vi "Lab Panel V6.00.vi"() -> ()   [LabVIEW 2017] (continued)
                          tunnel: w826 -> [_ w839]
                          tunnel: w824 -> [_ w838]
                          frame False {
                            w836 = FALSE
                            n593 = local write "RUN LAB01-1"(w836) -> ()
                            n594 = local write "run lab01-1"(w836) -> ()
                          }
                          frame True {
                            n595 = stacked-sequence {
                              seq-local: [w849 _ _ _ _] -> [_ w870 _ _ _]
                              tunnel: w848 -> [w854 _ _ _ _]
                              tunnel: w847 -> [w850 _ _ _ _]
                              tunnel: w846 -> [w864 _ _ _ _]
                              tunnel: w845 -> [w857 _ _ _ _]
                              tunnel: w844 -> [w852 _ _ _ _]
                              tunnel: [_ w871 _ _ _] -> w843
                              tunnel: w842 -> [_ _ _ w892 _]
                              tunnel: w841 -> [_ _ _ w902 _]
                              tunnel: w840 -> [_ _ _ w901 _]
                              tunnel: w839 -> [_ _ _ _ _]
                              tunnel: w838 -> [_ _ _ _ w908]
                              frame #0 {
                                w851 = "\\"
                                n596 = case shown="\"CHART TEST\", Default" w864 {
                                tunnel: ["L01-1-CHART TEST-" "L01-1-CYCLE TEST-" "L01-1-T-RISE TEST-"] -> w860
                                frame "CHART TEST", Default {
                                }
                                frame "CYCLE TEST" {
                                }
                                frame "T-RISE TEST" {
                                }
                                }
                                n597 = local read "SET LAB01-1"() -> (w859:T6)
                                n598 = Unbundle By Name(w859) -> ("DESCRIPTION"=w858:string)
                                n599 = Concatenate Strings(w854, "\\", w852, w851, w850, w851) -> (w861:string)
                                n600 = String To Path(string=w861) -> (path=w863:path)
                                n601 = Concatenate Strings(w861, w860, w858, "-", w857, ".tdms") -> (w849:string)
                                n602 = Create Folder(path (use dialog)=w863) -> (error out=w862:errorcluster)  [unwired: 2 in, 2 out]
                                n603 = call <vilib>:"Clear Errors.vi"("error in (no error)"=w862) -> ()  [unwired: 5 in, 2 out]
                                n604 = global write "Global 1.vi" "LAB01-1 FILE"(w849) -> ()
                              }
                              frame #1 {
                                (unwired) FALSE
                                n605 = String To Path(string=w870) -> (path=w868:path)
                                n606 = TDMS Open(6:FALSE, 10:T22."create or replace" ("operation (0:open)"), 11:w868) -> (0:w871:errorcluster, 3:→"TDMS LAB01-1":refnum<k34>)  [unwired: 4 in]
                              }
                              frame #2 {
                                n607 = local read "TDMS LAB01-1"() -> (w890:refnum<k34>)
                                n608 = local read "SET LAB01-1"() -> (w879:T6)
                                n609 = Build Array("Testers Name", "Description", "Set Test Cycles", "T-Rise minutes", "T-Rise Deg C") -> (w880:string[])
                                n610 = Unbundle(w879) -> ("NAME"=w878:string, "DESCRIPTION"=w877:string, "CYCLES"=w876:dbl, "T-RISE mins"=w875:dbl, "T-RISE deg C"=w874:dbl)
                                n611 = Number To Decimal String(number=w876) -> (decimal integer string=w889:string)  [unwired: 1 in]
                                n612 = Number To Decimal String(number=w875) -> (decimal integer string=w888:string)  [unwired: 1 in]
                                n613 = Number To Decimal String(number=w874) -> (decimal integer string=w887:string)  [unwired: 1 in]
                                n614 = Build Array(w878, w877, w889, w888, w887) -> (w886:string[])
                                n615 = TDMS Set Properties(5:w886, 7:w880, 11:w890) -> ()  [unwired: 3 in, 4 out]
                              }
                              frame #3 {
                                n616 = local read "DISP LAB01-1"() -> (w900:T4)
                                n617 = Concatenate Strings("LAB01-1  ", w892) -> (w891:string)
                                n618 = Two Button Dialog(message=w891, 1:w901, 2:w902) -> (T button?=w894:bool)
                                n619 = case shown="True" w894 {
                                tunnel: w900 -> [w905 w906]
                                tunnel: [w905 w906] -> w899
                                tunnel: [w904 w907] -> w898
                                tunnel: [w903 w907] -> w897
                                frame False {
                                n620 = Unbundle(w905) -> ("CYCLE"=w904:dbl, "MINS"=w903:dbl)  [unwired: 1 out]
                                }
                                frame True {
                                w907 = 0.0
                                }
                                }
                                n621 = Bundle(cluster=w899, "CYCLE"=w898, "MINS"=w897, "STATUS"="RUN") -> (w896:T4)
                                n622 = local write "DISP LAB01-1"(w896) -> ()
                              }
                              frame #4 {
                                n623 = local read "TEMP START LAB01-1"() -> (w910:cluster{"TL":dbl, "TN":dbl})
                                n624 = Bundle(cluster=w910, "TL"=w908, "TN"=w908) -> (w909:cluster{"TL":dbl, "TN":dbl})
                                n625 = local write "TEMP START LAB01-1"(w909) -> ()
                              }
                            }
                          }
                        }
                      }
                    }
                  }
                }
              }
              event "RUN LAB01-2": Value Change {
                n626 = event-data() -> ("NewVal"=w915:bool)  [unwired: 1 in, 5 out]
                n627 = local write "run lab01-2"(w915) -> ()
                n628 = case shown="True" w915 {
                  tunnel: w921 -> [_ w959]
                  tunnel: w920 -> [_ w958]
                  tunnel: w918 -> [w923 w957]
                  tunnel: w919 -> [_ w956]
                  tunnel: w917 -> [_ w955]
                  tunnel: [w922 w954] -> w916
                  tunnel: w914 -> [_ w953]
                  tunnel: w913 -> [_ w952]
                  tunnel: w912 -> [_ w951]
                  tunnel: w911 -> [_ w949]
                  frame False {
                    # "stop test"
                    n629 = stacked-sequence {
                      tunnel: w923 -> [w932 _]
                      tunnel: [w924 _] -> w922
                      frame #0 {
                        n630 = local read "DISP LAB01-2"() -> (w931:T4)
                        n631 = Unbundle(w931) -> ("CYCLE"=w929:dbl, "MINS"=w930:dbl)  [unwired: 1 out]
                        n632 = case shown="\"CHART TEST\", Default" w932 {
                          tunnel: w930 -> [_ _ w939]
                          tunnel: w929 -> [w937 w938 _]
                          tunnel: [w937 w938 w939] -> w928
                          frame "CHART TEST", Default {
                          }
                          frame "CYCLE TEST" {
                          }
                          frame "T-RISE TEST" {
                          }
                        }
                        n633 = local read "TDMS LAB01-2"() -> (w936:refnum<k34>)
                        n634 = Build Array("STOPPED") -> (w933:string[])
                        n635 = Build Array(w928) -> (w927:dbl[])
                        n636 = TDMS Write(0:w936, 5:"TEST RESULT", 7:w933, 9:w927) -> (4:w925:refnum<k34>, 15:w926:errorcluster)  [unwired: 2 in, 2 out]
                        n637 = TDMS Close(8:w926, 11:w925) -> (0:w924:errorcluster)  [unwired: 1 out]
                      }
                      frame #1 {
                        n638 = local read "DISP LAB01-2"() -> (w943:T4)
                        n639 = stacked-sequence {
                          tunnel: "LAB01-2" -> [w945 w947]
                          frame #0 {
                            n640 = call "sub vi - defrag tdms v1.vi"("panel id"=w945) -> ("error out"=w944:errorcluster)  [unwired: 10 in]
                            n641 = local write "data file error"(w944) -> ()
                          }
                          frame #1 {
                            n642 = call "Save data file (stop) v3.vi"("panel id"=w947) -> ("network file save error"=w946:errorcluster)  [unwired: 9 in, 1 out]
                            n643 = local write "RESULT LAB01-2"(FALSE) -> ()
                            n644 = local write "data file error"(w946) -> ()
                          }
                        }
                        n645 = Bundle(cluster=w943, "STATUS"="STOP") -> (w941:T4)  [unwired: 2 in]
                        n646 = local write "DISP LAB01-2"(w941) -> ()
                      }
                    }
                  }
                  frame True {
                    n647 = local read "SIG LAB01-2"() -> (w950:T2)
                    n648 = stacked-sequence {
                      seq-local: [w961 _] -> [_ w965]
                      tunnel: w959 -> [_ w975]
                      tunnel: w958 -> [_ w974]
                      tunnel: w957 -> [_ w973]
                      tunnel: w956 -> [_ w972]
                      tunnel: w955 -> [_ w971]
                      tunnel: [_ w970] -> w954
                      tunnel: w953 -> [_ w969]
                      tunnel: w952 -> [_ w968]
                      tunnel: w951 -> [_ w967]
                      tunnel: w950 -> [w960 w966]
                      tunnel: w949 -> [_ w964]
                      frame #0 {
                        n649 = Unbundle(w960) -> ("AMPS"=w963:dbl)  [unwired: 4 out]
                        n650 = call "Check For Amps on v1.vi"("ID"="LAB01-2", "amps"=w963) -> ("amps"=w961:bool)  [unwired: 9 in]
                      }
                      frame #1 {
                        n651 = case shown="True" w965 {
                          tunnel: w975 -> [_ w988]
                          tunnel: w974 -> [_ w987]
                          tunnel: w973 -> [_ w986]
                          tunnel: w972 -> [_ w985]
                          tunnel: w971 -> [_ w984]
                          tunnel: [errorcluster {"status"=FALSE, "code"=0, "source"=""} ("error out") w983] -> w970
                          tunnel: w969 -> [_ w982]
                          tunnel: w968 -> [_ w981]
                          tunnel: w967 -> [_ w980]
                          tunnel: w966 -> [_ w979]
                          tunnel: w964 -> [_ w978]
                          frame False {
                            w976 = FALSE
                            n652 = local write "RUN LAB01-2"(w976) -> ()
                            n653 = local write "run lab01-2"(w976) -> ()
                          }
                          frame True {
                            n654 = stacked-sequence {
                              seq-local: [w989 _ _ _ _] -> [_ w1013 _ _ _]
                              tunnel: w988 -> [w994 _ _ _ _]
                              tunnel: w987 -> [w991 _ _ _ _]
                              tunnel: w986 -> [w1004 _ _ _ _]
                              tunnel: w985 -> [w997 _ _ _ _]
                              tunnel: w984 -> [w992 _ _ _ _]
                              tunnel: [_ w1008 _ _ _] -> w983
                              tunnel: w982 -> [_ _ _ w1035 _]
                              tunnel: w981 -> [_ _ _ w1034 _]
                              tunnel: w980 -> [_ _ _ w1033 _]
                              tunnel: w979 -> [_ _ _ _ _]
                              tunnel: w978 -> [_ _ _ _ w1048]
                              frame #0 {
                                w990 = "\\"
                                n655 = local read "SET LAB01-2"() -> (w999:T5)
                                n656 = case shown="\"CYCLE TEST\"" w1004 {
                                tunnel: ["L01-2-CHART TEST-" "L01-2-CYCLE TEST-" "L01-2-T-RISE TEST-"] -> w1000
                                frame "CHART TEST", Default {
                                }
                                frame "CYCLE TEST" {
                                }
                                frame "T-RISE TEST" {
                                }
                                }
                                n657 = Unbundle(w999) -> ("DESCRIPTION"=w998:string)  [unwired: 4 out]
                                n658 = Concatenate Strings(w994, "\\", w992, w990, w991, w990) -> (w1001:string)
                                n659 = String To Path(string=w1001) -> (path=w1003:path)
                                n660 = Concatenate Strings(w1001, w1000, w998, "-", w997, ".tdms") -> (w989:string)
                                n661 = Create Folder(path (use dialog)=w1003) -> (error out=w1002:errorcluster)  [unwired: 2 in, 2 out]
                                n662 = call <vilib>:"Clear Errors.vi"("error in (no error)"=w1002) -> ()  [unwired: 5 in, 2 out]
                                n663 = global write "Global 1.vi" "LAB01-2 FILE"(w989) -> ()
                              }
                              frame #1 {
                                (unwired) FALSE
                                n664 = String To Path(string=w1013) -> (path=w1009:path)
                                n665 = TDMS Open(6:FALSE, 10:T22."create or replace" ("operation (0:open)"), 11:w1009) -> (0:w1008:errorcluster, 3:→"TDMS LAB01-2":refnum<k34>)  [unwired: 4 in]
                              }
                              frame #2 {
                                n666 = local read "SET LAB01-2"() -> (w1019:T5)
                                n667 = local read "TDMS LAB01-2"() -> (w1030:refnum<k34>)
                                n668 = Build Array("Testers Name", "Description", "Set Test Cycles", "T-Rise minutes", "T-Rise Deg C") -> (w1020:string[])
                                n669 = Unbundle(w1019) -> ("NAME"=w1018:string, "DESCRIPTION"=w1017:string, "CYCLES"=w1016:dbl, "T-RISE mins"=w1015:dbl, "T-RISE deg C"=w1014:dbl)
                                n670 = Number To Decimal String(number=w1016) -> (decimal integer string=w1029:string)  [unwired: 1 in]
                                n671 = Number To Decimal String(number=w1015) -> (decimal integer string=w1028:string)  [unwired: 1 in]
                                n672 = Number To Decimal String(number=w1014) -> (decimal integer string=w1027:string)  [unwired: 1 in]
                                n673 = Build Array(w1018, w1017, w1029, w1028, w1027) -> (w1026:string[])
                                n674 = TDMS Set Properties(5:w1026, 7:w1020, 11:w1030) -> ()  [unwired: 3 in, 4 out]
                              }
                              frame #3 {
                                n675 = local read "DISP LAB01-2"() -> (w1032:T4)
                                n676 = Concatenate Strings("LAB01-2  ", w1035) -> (w1036:string)
                                n677 = Two Button Dialog(message=w1036, 1:w1033, 2:w1034) -> (T button?=w1038:bool)
                                n678 = case shown="True" w1038 {
                                tunnel: w1032 -> [w1045 w1046]
                                tunnel: [w1045 w1046] -> w1042
                                tunnel: [w1044 w1047] -> w1041
                                tunnel: [w1043 w1047] -> w1040
                                frame False {
                                n679 = Unbundle(w1045) -> ("CYCLE"=w1044:dbl, "MINS"=w1043:dbl)  [unwired: 1 out]
                                }
                                frame True {
                                w1047 = 0.0
                                }
                                }
                                n680 = Bundle(cluster=w1042, "CYCLE"=w1041, "MINS"=w1040, "STATUS"="RUN") -> (w1031:T4)
                                n681 = local write "DISP LAB01-2"(w1031) -> ()
                              }
                              frame #4 {
                                n682 = local read "TEMP START LAB01-2"() -> (w1050:cluster{"TL":dbl, "TN":dbl})
                                n683 = Bundle(cluster=w1050, "TL"=w1048, "TN"=w1048) -> (w1049:cluster{"TL":dbl, "TN":dbl})
                                n684 = local write "TEMP START LAB01-2"(w1049) -> ()
                              }
                            }
                          }
                        }
                      }
                    }
                  }
                }
              }
              event "RUN LAB02-1": Value Change {
                n685 = event-data() -> ("NewVal"=w1056:bool)  [unwired: 1 in, 5 out]
                n686 = local read "SIG LAB02-1"() -> (w1052:T2)
                n687 = case shown="True" w1056 {
                  tunnel: w1062 -> [_ w1100]
                  tunnel: w1061 -> [_ w1099]
                  tunnel: w1059 -> [w1064 w1098]
                  tunnel: w1060 -> [_ w1097]
                  tunnel: w1058 -> [_ w1096]
                  tunnel: [w1063 w1095] -> w1057
                  tunnel: w1055 -> [_ w1094]
                  tunnel: w1054 -> [_ w1093]
                  tunnel: w1053 -> [_ w1092]
                  tunnel: w1052 -> [_ w1091]
                  tunnel: w1051 -> [_ w1090]
                  frame False {
                    # "stop test"
                    n688 = stacked-sequence {
                      tunnel: w1064 -> [w1073 _]
                      tunnel: [w1065 _] -> w1063
                      frame #0 {
                        n689 = local read "DISP LAB02-1"() -> (w1072:T4)
                        n690 = Unbundle(w1072) -> ("CYCLE"=w1070:dbl, "MINS"=w1071:dbl)  [unwired: 1 out]
                        n691 = case shown="\"CYCLE TEST\"" w1073 {
                          tunnel: w1071 -> [_ _ w1080]
                          tunnel: w1070 -> [w1078 w1079 _]
                          tunnel: [w1078 w1079 w1080] -> w1069
                          frame "CHART TEST", Default {
                          }
                          frame "CYCLE TEST" {
                          }
                          frame "T-RISE TEST" {
                          }
                        }
                        n692 = local read "TDMS LAB02-1"() -> (w1077:refnum<k34>)
                        n693 = Build Array("STOPPED") -> (w1074:string[])
                        n694 = Build Array(w1069) -> (w1068:dbl[])
                        n695 = TDMS Write(0:w1077, 5:"TEST RESULT", 7:w1074, 9:w1068) -> (4:w1066:refnum<k34>, 15:w1067:errorcluster)  [unwired: 2 in, 2 out]
                        n696 = TDMS Close(8:w1067, 11:w1066) -> (0:w1065:errorcluster)  [unwired: 1 out]
                      }
                      frame #1 {
                        n697 = local read "DISP LAB02-1"() -> (w1084:T4)
                        n698 = stacked-sequence {
                          tunnel: "LAB02-1" -> [w1086 w1088]
                          frame #0 {
                            n699 = call "sub vi - defrag tdms v1.vi"("panel id"=w1086) -> ("error out"=w1085:errorcluster)  [unwired: 10 in]
                            n700 = local write "data file error"(w1085) -> ()
                          }
                          frame #1 {
                            n701 = local write "RESULT LAB02-1"(FALSE) -> ()
                            n702 = call "Save data file (stop) v3.vi"("panel id"=w1088) -> ("network file save error"=w1087:errorcluster)  [unwired: 9 in, 1 out]
                            n703 = local write "data file error"(w1087) -> ()
                          }
                        }
                        n704 = Bundle(cluster=w1084, "STATUS"="STOP") -> (w1082:T4)  [unwired: 2 in]
                        n705 = local write "DISP LAB02-1"(w1082) -> ()
                      }
                    }
                  }
                  frame True {
                    n706 = stacked-sequence {
                      seq-local: [w1102 _] -> [_ w1106]
                      tunnel: w1100 -> [_ w1116]
                      tunnel: w1099 -> [_ w1115]
                      tunnel: w1098 -> [_ w1114]
                      tunnel: w1097 -> [_ w1113]
                      tunnel: w1096 -> [_ w1112]
                      tunnel: [_ w1111] -> w1095
                      tunnel: w1094 -> [_ w1110]
                      tunnel: w1093 -> [_ w1109]
                      tunnel: w1092 -> [_ w1108]
                      tunnel: w1091 -> [w1101 w1107]
                      tunnel: w1090 -> [_ w1105]
                      frame #0 {
                        n707 = Unbundle(w1101) -> ("AMPS"=w1104:dbl)  [unwired: 4 out]
                        n708 = call "Check For Amps on v1.vi"("ID"="LAB02-1", "amps"=w1104) -> ("amps"=w1102:bool)  [unwired: 9 in]
                      }
                      frame #1 {
                        n709 = case shown="True" w1106 {
                          tunnel: w1116 -> [_ w1129]
                          tunnel: w1115 -> [_ w1128]
                          tunnel: w1114 -> [_ w1127]
                          tunnel: w1113 -> [_ w1126]
                          tunnel: w1112 -> [_ w1125]
                          tunnel: [errorcluster {"status"=FALSE, "code"=0, "source"=""} ("error out") w1124] -> w1111
                          tunnel: w1110 -> [_ w1123]
                          tunnel: w1109 -> [_ w1122]
                          tunnel: w1108 -> [_ w1121]
                          tunnel: w1107 -> [_ w1120]
                          tunnel: w1105 -> [_ w1119]
                          frame False {
                            w1118 = FALSE
                            n710 = local write "RUN LAB02-1"(w1118) -> ()
                            n711 = local write "run lab02-1"(w1118) -> ()
                          }
                          frame True {
                            n712 = stacked-sequence {
                              seq-local: [w1130 _ _ _ _] -> [_ w1154 _ _ _]
                              tunnel: w1129 -> [w1135 _ _ _ _]
                              tunnel: w1128 -> [w1132 _ _ _ _]
                              tunnel: w1127 -> [w1145 _ _ _ _]
                              tunnel: w1126 -> [w1138 _ _ _ _]
                              tunnel: w1125 -> [w1133 _ _ _ _]
                              tunnel: [_ w1149 _ _ _] -> w1124
                              tunnel: w1123 -> [_ _ _ w1175 _]
                              tunnel: w1122 -> [_ _ _ w1174 _]
                              tunnel: w1121 -> [_ _ _ w1173 _]
                              tunnel: w1120 -> [_ _ _ _ _]
                              tunnel: w1119 -> [_ _ _ _ w1189]
                              frame #0 {
                                w1131 = "\\"
                                n713 = local read "SET LAB02-1"() -> (w1140:T5)
                                n714 = case shown="\"CYCLE TEST\"" w1145 {
                                tunnel: ["L02-1-CHART TEST-" "L02-1-CYCLE TEST-" "L02-1-T-RISE TEST-"] -> w1141
                                frame "CHART TEST", Default {
                                }
                                frame "CYCLE TEST" {
                                }
                                frame "T-RISE TEST" {
                                }
                                }
                                n715 = Unbundle(w1140) -> ("DESCRIPTION"=w1139:string)  [unwired: 4 out]
                                n716 = Concatenate Strings(w1135, "\\", w1133, w1131, w1132, w1131) -> (w1142:string)
                                n717 = String To Path(string=w1142) -> (path=w1144:path)
                                n718 = Concatenate Strings(w1142, w1141, w1139, "-", w1138, ".tdms") -> (w1130:string)
                                n719 = Create Folder(path (use dialog)=w1144) -> (error out=w1143:errorcluster)  [unwired: 2 in, 2 out]
                                n720 = global write "Global 1.vi" "LAB02-1 FILE"(w1130) -> ()
                                n721 = call <vilib>:"Clear Errors.vi"("error in (no error)"=w1143) -> ()  [unwired: 5 in, 2 out]
                              }
                              frame #1 {
                                (unwired) FALSE
                                n722 = String To Path(string=w1154) -> (path=w1150:path)
                                n723 = TDMS Open(6:FALSE, 10:T22."create or replace" ("operation (0:open)"), 11:w1150) -> (0:w1149:errorcluster, 3:→"TDMS LAB02-1":refnum<k34>)  [unwired: 4 in]
                              }
                              frame #2 {
                                n724 = local read "SET LAB02-1"() -> (w1160:T5)
                                n725 = local read "TDMS LAB02-1"() -> (w1171:refnum<k34>)
                                n726 = Build Array("Testers Name", "Description", "Set Test Cycles", "T-Rise minutes", "T-Rise Deg C") -> (w1161:string[])
                                n727 = Unbundle(w1160) -> ("NAME"=w1159:string, "DESCRIPTION"=w1158:string, "CYCLES"=w1157:dbl, "T-RISE mins"=w1156:dbl, "T-RISE deg C"=w1155:dbl)
                                n728 = Number To Decimal String(number=w1157) -> (decimal integer string=w1170:string)  [unwired: 1 in]
                                n729 = Number To Decimal String(number=w1156) -> (decimal integer string=w1169:string)  [unwired: 1 in]
                                n730 = Number To Decimal String(number=w1155) -> (decimal integer string=w1168:string)  [unwired: 1 in]
                                n731 = Build Array(w1159, w1158, w1170, w1169, w1168) -> (w1167:string[])
                                n732 = TDMS Set Properties(5:w1167, 7:w1161, 11:w1171) -> ()  [unwired: 3 in, 4 out]
                              }
                              frame #3 {
                                n733 = local read "DISP LAB02-1"() -> (w1176:T4)
                                n734 = Concatenate Strings("LAB02-1  ", w1175) -> (w1177:string)
                                n735 = Two Button Dialog(message=w1177, 1:w1173, 2:w1174) -> (T button?=w1179:bool)
                                n736 = case shown="True" w1179 {
                                tunnel: w1176 -> [w1186 w1187]
                                tunnel: [w1186 w1187] -> w1183
                                tunnel: [w1185 w1188] -> w1182
                                tunnel: [w1184 w1188] -> w1181
                                frame False {
                                n737 = Unbundle(w1186) -> ("CYCLE"=w1185:dbl, "MINS"=w1184:dbl)  [unwired: 1 out]
                                }
                                frame True {
                                w1188 = 0.0
                                }
                                }
                                n738 = Bundle(cluster=w1183, "CYCLE"=w1182, "MINS"=w1181, "STATUS"="RUN") -> (w1172:T4)
                                n739 = local write "DISP LAB02-1"(w1172) -> ()
                              }
                              frame #4 {
                                n740 = local read "TEMP START LAB02-1"() -> (w1191:cluster{"TL":dbl, "TN":dbl})
                                n741 = Bundle(cluster=w1191, "TL"=w1189, "TN"=w1189) -> (w1190:cluster{"TL":dbl, "TN":dbl})
                                n742 = local write "TEMP START LAB02-1"(w1190) -> ()
                              }
                            }
                          }
                        }
                      }
                    }
                  }
                }
                n743 = local write "run lab02-1"(w1056) -> ()
              }
              event "RUN LAB02-2": Value Change {
                n744 = event-data() -> ("NewVal"=w1196:bool)  [unwired: 1 in, 5 out]
                n745 = local write "run lab02-2"(w1196) -> ()
                n746 = case shown="True" w1196 {
                  tunnel: w1202 -> [_ w1240]
                  tunnel: w1201 -> [_ w1239]
                  tunnel: w1199 -> [w1204 w1238]
                  tunnel: w1200 -> [_ w1237]
                  tunnel: w1198 -> [_ w1236]
                  tunnel: [w1203 w1235] -> w1197
                  tunnel: w1195 -> [_ w1234]
                  tunnel: w1194 -> [_ w1233]
                  tunnel: w1193 -> [_ w1232]
                  tunnel: w1192 -> [_ w1230]
                  frame False {
                    # "stop test"
                    n747 = stacked-sequence {
                      tunnel: w1204 -> [w1213 _]
                      tunnel: [w1205 _] -> w1203
                      frame #0 {
                        n748 = local read "DISP LAB02-2"() -> (w1212:T4)
                        n749 = Unbundle(w1212) -> ("CYCLE"=w1210:dbl, "MINS"=w1211:dbl)  [unwired: 1 out]
                        n750 = case shown="\"CYCLE TEST\"" w1213 {
                          tunnel: w1211 -> [_ _ w1220]
                          tunnel: w1210 -> [w1218 w1219 _]
                          tunnel: [w1218 w1219 w1220] -> w1209
                          frame "CHART TEST", Default {
                          }
                          frame "CYCLE TEST" {
                          }
                          frame "T-RISE TEST" {
                          }
                        }
                        n751 = local read "TDMS LAB02-2"() -> (w1217:refnum<k34>)
                        n752 = Build Array("STOPPED") -> (w1214:string[])
                        n753 = Build Array(w1209) -> (w1208:dbl[])
                        n754 = TDMS Write(0:w1217, 5:"TEST RESULT", 7:w1214, 9:w1208) -> (4:w1206:refnum<k34>, 15:w1207:errorcluster)  [unwired: 2 in, 2 out]
                        n755 = TDMS Close(8:w1207, 11:w1206) -> (0:w1205:errorcluster)  [unwired: 1 out]
                      }
                      frame #1 {
                        n756 = local read "DISP LAB02-2"() -> (w1224:T4)
                        n757 = stacked-sequence {
                          tunnel: "LAB02-2" -> [w1226 w1228]
                          frame #0 {
                            n758 = call "sub vi - defrag tdms v1.vi"("panel id"=w1226) -> ("error out"=w1225:errorcluster)  [unwired: 10 in]
                            n759 = local write "data file error"(w1225) -> ()
                          }
                          frame #1 {
                            n760 = call "Save data file (stop) v3.vi"("panel id"=w1228) -> ("network file save error"=w1227:errorcluster)  [unwired: 9 in, 1 out]
                            n761 = local write "RESULT LAB02-2"(FALSE) -> ()
                            n762 = local write "data file error"(w1227) -> ()
                          }
                        }
                        n763 = Bundle(cluster=w1224, "STATUS"="STOP") -> (w1222:T4)  [unwired: 2 in]
                        n764 = local write "DISP LAB02-2"(w1222) -> ()
                      }
                    }
                  }
                  frame True {
                    n765 = local read "SIG LAB02-2"() -> (w1231:T2)
                    n766 = stacked-sequence {
                      seq-local: [w1242 _] -> [_ w1246]
                      tunnel: w1240 -> [_ w1256]
                      tunnel: w1239 -> [_ w1255]
                      tunnel: w1238 -> [_ w1254]
                      tunnel: w1237 -> [_ w1253]
                      tunnel: w1236 -> [_ w1252]
                      tunnel: [_ w1251] -> w1235
                      tunnel: w1234 -> [_ w1250]
                      tunnel: w1233 -> [_ w1249]
                      tunnel: w1232 -> [_ w1248]
                      tunnel: w1231 -> [w1241 w1247]
                      tunnel: w1230 -> [_ w1245]
                      frame #0 {
                        n767 = Unbundle(w1241) -> ("AMPS"=w1244:dbl)  [unwired: 4 out]
                        n768 = call "Check For Amps on v1.vi"("ID"="LAB02-2", "amps"=w1244) -> ("amps"=w1242:bool)  [unwired: 9 in]
                      }
                      frame #1 {
                        n769 = case shown="True" w1246 {
                          tunnel: w1256 -> [_ w1269]
                          tunnel: w1255 -> [_ w1268]
                          tunnel: w1254 -> [_ w1267]
                          tunnel: w1253 -> [_ w1266]
                          tunnel: w1252 -> [_ w1265]
                          tunnel: [errorcluster {"status"=FALSE, "code"=0, "source"=""} ("error out") w1264] -> w1251
                          tunnel: w1250 -> [_ w1263]
                          tunnel: w1249 -> [_ w1262]
                          tunnel: w1248 -> [_ w1261]
                          tunnel: w1247 -> [_ w1260]
                          tunnel: w1245 -> [_ w1259]
                          frame False {
                            w1257 = FALSE
                            n770 = local write "RUN LAB02-2"(w1257) -> ()
                            n771 = local write "run lab02-2"(w1257) -> ()
                          }
                          frame True {
                            n772 = stacked-sequence {
                              seq-local: [w1270 _ _ _ _] -> [_ w1294 _ _ _]
                              tunnel: w1269 -> [w1275 _ _ _ _]
                              tunnel: w1268 -> [w1272 _ _ _ _]
                              tunnel: w1267 -> [w1285 _ _ _ _]
                              tunnel: w1266 -> [w1278 _ _ _ _]
                              tunnel: w1265 -> [w1273 _ _ _ _]
                              tunnel: [_ w1289 _ _ _] -> w1264
                              tunnel: w1263 -> [_ _ _ w1315 _]
                              tunnel: w1262 -> [_ _ _ w1314 _]
                              tunnel: w1261 -> [_ _ _ w1313 _]
                              tunnel: w1260 -> [_ _ _ _ _]
                              tunnel: w1259 -> [_ _ _ _ w1329]
                              frame #0 {
                                w1271 = "\\"
                                n773 = local read "SET LAB02-2"() -> (w1280:T5)
                                n774 = case shown="\"CYCLE TEST\"" w1285 {
                                tunnel: ["L02-2-CHART TEST-" "L02-2-CYCLE TEST-" "L02-2-T-RISE TEST-"] -> w1281
                                frame "CHART TEST", Default {
                                }
                                frame "CYCLE TEST" {
                                }
                                frame "T-RISE TEST" {
                                }
                                }
                                n775 = Unbundle(w1280) -> ("DESCRIPTION"=w1279:string)  [unwired: 4 out]
                                n776 = Concatenate Strings(w1275, "\\", w1273, w1271, w1272, w1271) -> (w1282:string)
                                n777 = String To Path(string=w1282) -> (path=w1284:path)
                                n778 = Concatenate Strings(w1282, w1281, w1279, "-", w1278, ".tdms") -> (w1270:string)
                                n779 = Create Folder(path (use dialog)=w1284) -> (error out=w1283:errorcluster)  [unwired: 2 in, 2 out]
                                n780 = global write "Global 1.vi" "LAB02-2 FILE"(w1270) -> ()
                                n781 = call <vilib>:"Clear Errors.vi"("error in (no error)"=w1283) -> ()  [unwired: 5 in, 2 out]
                              }
                              frame #1 {
                                (unwired) FALSE
                                n782 = String To Path(string=w1294) -> (path=w1290:path)
                                n783 = TDMS Open(6:FALSE, 10:T22."create or replace" ("operation (0:open)"), 11:w1290) -> (0:w1289:errorcluster, 3:→"TDMS LAB02-2":refnum<k34>)  [unwired: 4 in]
                              }
                              frame #2 {
                                n784 = local read "SET LAB02-2"() -> (w1300:T5)
                                n785 = local read "TDMS LAB02-2"() -> (w1311:refnum<k34>)
                                n786 = Build Array("Testers Name", "Description", "Set Test Cycles", "T-Rise minutes", "T-Rise Deg C") -> (w1301:string[])
                                n787 = Unbundle(w1300) -> ("NAME"=w1299:string, "DESCRIPTION"=w1298:string, "CYCLES"=w1297:dbl, "T-RISE mins"=w1296:dbl, "T-RISE deg C"=w1295:dbl)
                                n788 = Number To Decimal String(number=w1297) -> (decimal integer string=w1310:string)  [unwired: 1 in]
                                n789 = Number To Decimal String(number=w1296) -> (decimal integer string=w1309:string)  [unwired: 1 in]
                                n790 = Number To Decimal String(number=w1295) -> (decimal integer string=w1308:string)  [unwired: 1 in]
                                n791 = Build Array(w1299, w1298, w1310, w1309, w1308) -> (w1307:string[])
                                n792 = TDMS Set Properties(5:w1307, 7:w1301, 11:w1311) -> ()  [unwired: 3 in, 4 out]
                              }
                              frame #3 {
                                n793 = local read "DISP LAB02-2"() -> (w1316:T4)
                                n794 = Concatenate Strings("LAB02-2  ", w1315) -> (w1317:string)
                                n795 = Two Button Dialog(message=w1317, 1:w1313, 2:w1314) -> (T button?=w1319:bool)
                                n796 = case shown="True" w1319 {
                                tunnel: w1316 -> [w1326 w1327]
                                tunnel: [w1326 w1327] -> w1323
                                tunnel: [w1325 w1328] -> w1322
                                tunnel: [w1324 w1328] -> w1321
                                frame False {
                                n797 = Unbundle(w1326) -> ("CYCLE"=w1325:dbl, "MINS"=w1324:dbl)  [unwired: 1 out]
                                }
                                frame True {
                                w1328 = 0.0
                                }
                                }
                                n798 = Bundle(cluster=w1323, "CYCLE"=w1322, "MINS"=w1321, "STATUS"="RUN") -> (w1312:T4)
                                n799 = local write "DISP LAB02-2"(w1312) -> ()
                              }
                              frame #4 {
                                n800 = local read "TEMP START LAB02-2"() -> (w1331:cluster{"TL":dbl, "TN":dbl})
                                n801 = Bundle(cluster=w1331, "TL"=w1329, "TN"=w1329) -> (w1330:cluster{"TL":dbl, "TN":dbl})
                                n802 = local write "TEMP START LAB02-2"(w1330) -> ()
                              }
                            }
                          }
                        }
                      }
                    }
                  }
                }
              }
              event "RUN LAB03-1": Value Change {
                n803 = event-data() -> ("NewVal"=w1336:bool)  [unwired: 1 in, 5 out]
                n804 = local write "run lab03-1"(w1336) -> ()
                n805 = case shown="True" w1336 {
                  tunnel: w1342 -> [_ w1380]
                  tunnel: w1341 -> [_ w1379]
                  tunnel: w1339 -> [w1344 w1378]
                  tunnel: w1340 -> [_ w1377]
                  tunnel: w1338 -> [_ w1376]
                  tunnel: [w1343 w1375] -> w1337
                  tunnel: w1335 -> [_ w1374]
                  tunnel: w1334 -> [_ w1373]
                  tunnel: w1333 -> [_ w1372]
                  tunnel: w1332 -> [_ w1370]
                  frame False {
                    # "stop test"
                    n806 = stacked-sequence {
                      tunnel: w1344 -> [w1353 _]
                      tunnel: [w1345 _] -> w1343
                      frame #0 {
                        n807 = local read "DISP LAB03-1"() -> (w1352:T4)
                        n808 = Unbundle(w1352) -> ("CYCLE"=w1350:dbl, "MINS"=w1351:dbl)  [unwired: 1 out]
                        n809 = case shown="\"CYCLE TEST\"" w1353 {
                          tunnel: w1351 -> [_ _ w1360]
                          tunnel: w1350 -> [w1358 w1359 _]
                          tunnel: [w1358 w1359 w1360] -> w1349
                          frame "CHART TEST", Default {
                          }
                          frame "CYCLE TEST" {
                          }
                          frame "T-RISE TEST" {
                          }
                        }
                        n810 = local read "TDMS LAB03-1"() -> (w1357:refnum<k34>)
                        n811 = Build Array("STOPPED") -> (w1354:string[])
                        n812 = Build Array(w1349) -> (w1348:dbl[])
                        n813 = TDMS Write(0:w1357, 5:"TEST RESULT", 7:w1354, 9:w1348) -> (4:w1346:refnum<k34>, 15:w1347:errorcluster)  [unwired: 2 in, 2 out]
                        n814 = TDMS Close(8:w1347, 11:w1346) -> (0:w1345:errorcluster)  [unwired: 1 out]
                      }
                      frame #1 {
                        n815 = local read "DISP LAB03-1"() -> (w1364:T4)
                        n816 = stacked-sequence {
                          tunnel: "LAB03-1" -> [w1366 w1368]
                          frame #0 {
                            n817 = call "sub vi - defrag tdms v1.vi"("panel id"=w1366) -> ("error out"=w1365:errorcluster)  [unwired: 10 in]
                            n818 = local write "data file error"(w1365) -> ()
                          }
                          frame #1 {
                            n819 = call "Save data file (stop) v3.vi"("panel id"=w1368) -> ("network file save error"=w1367:errorcluster)  [unwired: 9 in, 1 out]
                            n820 = local write "RESULT LAB03-1"(FALSE) -> ()
                            n821 = local write "data file error"(w1367) -> ()
                          }
                        }
                        n822 = Bundle(cluster=w1364, "STATUS"="STOP") -> (w1362:T4)  [unwired: 2 in]
                        n823 = local write "DISP LAB03-1"(w1362) -> ()
                      }
                    }
                  }
                  frame True {
                    n824 = local read "SIG LAB03-1"() -> (w1371:T2)
                    n825 = stacked-sequence {
                      seq-local: [w1382 _] -> [_ w1386]
                      tunnel: w1380 -> [_ w1396]
                      tunnel: w1379 -> [_ w1395]
                      tunnel: w1378 -> [_ w1394]
                      tunnel: w1377 -> [_ w1393]
                      tunnel: w1376 -> [_ w1392]
                      tunnel: [_ w1391] -> w1375
                      tunnel: w1374 -> [_ w1390]
                      tunnel: w1373 -> [_ w1389]
                      tunnel: w1372 -> [_ w1388]
                      tunnel: w1371 -> [w1381 w1387]
                      tunnel: w1370 -> [_ w1385]
                      frame #0 {
                        n826 = Unbundle(w1381) -> ("AMPS"=w1384:dbl)  [unwired: 4 out]
                        n827 = call "Check For Amps on v1.vi"("ID"="LAB03-1", "amps"=w1384) -> ("amps"=w1382:bool)  [unwired: 9 in]
                      }
                      frame #1 {
                        n828 = case shown="True" w1386 {
                          tunnel: w1396 -> [_ w1409]
                          tunnel: w1395 -> [_ w1408]
                          tunnel: w1394 -> [_ w1407]
                          tunnel: w1393 -> [_ w1406]
                          tunnel: w1392 -> [_ w1405]
                          tunnel: [errorcluster {"status"=FALSE, "code"=0, "source"=""} ("error out") w1404] -> w1391
                          tunnel: w1390 -> [_ w1403]
                          tunnel: w1389 -> [_ w1402]
                          tunnel: w1388 -> [_ w1401]
                          tunnel: w1387 -> [_ w1400]
                          tunnel: w1385 -> [_ w1399]
                          frame False {
                            w1397 = FALSE
                            n829 = local write "RUN LAB03-1"(w1397) -> ()
                            n830 = local write "run lab03-1"(w1397) -> ()
                          }
                          frame True {
                            n831 = stacked-sequence {
                              seq-local: [w1410 _ _ _ _] -> [_ w1434 _ _ _]
                              tunnel: w1409 -> [w1415 _ _ _ _]
                              tunnel: w1408 -> [w1412 _ _ _ _]
                              tunnel: w1407 -> [w1425 _ _ _ _]
                              tunnel: w1406 -> [w1418 _ _ _ _]
                              tunnel: w1405 -> [w1413 _ _ _ _]
                              tunnel: [_ w1429 _ _ _] -> w1404
                              tunnel: w1403 -> [_ _ _ w1454 _]
                              tunnel: w1402 -> [_ _ _ w1453 _]
                              tunnel: w1401 -> [_ _ _ w1452 _]
                              tunnel: w1400 -> [_ _ _ _ _]
                              tunnel: w1399 -> [_ _ _ _ w1469]
                              frame #0 {
                                w1411 = "\\"
                                n832 = local read "SET LAB03-1"() -> (w1420:T5)
                                n833 = case shown="\"T-RISE TEST\"" w1425 {
                                tunnel: ["L03-1-CHART TEST-" "L03-1-CYCLE TEST-" "L03-1-T-RISE TEST-"] -> w1421
                                frame "CHART TEST", Default {
                                }
                                frame "CYCLE TEST" {
                                }
                                frame "T-RISE TEST" {
                                }
                                }
                                n834 = Unbundle(w1420) -> ("DESCRIPTION"=w1419:string)  [unwired: 4 out]
                                n835 = Concatenate Strings(w1415, "\\", w1413, w1411, w1412, w1411) -> (w1422:string)
                                n836 = String To Path(string=w1422) -> (path=w1424:path)
                                n837 = Concatenate Strings(w1422, w1421, w1419, "-", w1418, ".tdms") -> (w1410:string)
                                n838 = Create Folder(path (use dialog)=w1424) -> (error out=w1423:errorcluster)  [unwired: 2 in, 2 out]
                                n839 = global write "Global 1.vi" "LAB03-1 FILE"(w1410) -> ()
                                n840 = call <vilib>:"Clear Errors.vi"("error in (no error)"=w1423) -> ()  [unwired: 5 in, 2 out]
                              }
                              frame #1 {
                                (unwired) FALSE
                                n841 = String To Path(string=w1434) -> (path=w1430:path)
                                n842 = TDMS Open(6:FALSE, 10:T22."create or replace" ("operation (0:open)"), 11:w1430) -> (0:w1429:errorcluster, 3:→"TDMS LAB03-1":refnum<k34>)  [unwired: 4 in]
                              }
                              frame #2 {
                                n843 = local read "SET LAB03-1"() -> (w1440:T5)
                                n844 = local read "TDMS LAB03-1"() -> (w1451:refnum<k34>)
                                n845 = Build Array("Testers Name", "Description", "Set Test Cycles", "T-Rise minutes", "T-Rise Deg C") -> (w1441:string[])
                                n846 = Unbundle(w1440) -> ("NAME"=w1439:string, "DESCRIPTION"=w1438:string, "CYCLES"=w1437:dbl, "T-RISE mins"=w1436:dbl, "T-RISE deg C"=w1435:dbl)
                                n847 = Number To Decimal String(number=w1437) -> (decimal integer string=w1450:string)  [unwired: 1 in]
                                n848 = Number To Decimal String(number=w1436) -> (decimal integer string=w1449:string)  [unwired: 1 in]
                                n849 = Number To Decimal String(number=w1435) -> (decimal integer string=w1448:string)  [unwired: 1 in]
                                n850 = Build Array(w1439, w1438, w1450, w1449, w1448) -> (w1447:string[])
                                n851 = TDMS Set Properties(5:w1447, 7:w1441, 11:w1451) -> ()  [unwired: 3 in, 4 out]
                              }
                              frame #3 {
                                n852 = local read "DISP LAB03-1"() -> (w1456:T4)
                                n853 = Concatenate Strings("LAB03-1  ", w1454) -> (w1457:string)
                                n854 = Two Button Dialog(message=w1457, 1:w1452, 2:w1453) -> (T button?=w1459:bool)
                                n855 = case shown="True" w1459 {
                                tunnel: w1456 -> [w1466 w1467]
                                tunnel: [w1466 w1467] -> w1463
                                tunnel: [w1465 w1468] -> w1462
                                tunnel: [w1464 w1468] -> w1461
                                frame False {
                                n856 = Unbundle(w1466) -> ("CYCLE"=w1465:dbl, "MINS"=w1464:dbl)  [unwired: 1 out]
                                }
                                frame True {
                                w1468 = 0.0
                                }
                                }
                                n857 = Bundle(cluster=w1463, "CYCLE"=w1462, "MINS"=w1461, "STATUS"="RUN") -> (w1455:T4)
                                n858 = local write "DISP LAB03-1"(w1455) -> ()
                              }
                              frame #4 {
                                n859 = local read "TEMP START LAB03-1"() -> (w1471:cluster{"TL":dbl, "TN":dbl})
                                n860 = Bundle(cluster=w1471, "TL"=w1469, "TN"=w1469) -> (w1470:cluster{"TL":dbl, "TN":dbl})
                                n861 = local write "TEMP START LAB03-1"(w1470) -> ()
                              }
                            }
                          }
                        }
                      }
                    }
                  }
                }
              }
              event "RUN LAB03-2": Value Change {
                n862 = event-data() -> ("NewVal"=w1476:bool)  [unwired: 1 in, 5 out]
                n863 = local write "run lab03-2"(w1476) -> ()
                n864 = case shown="True" w1476 {
                  tunnel: w1482 -> [_ w1520]
                  tunnel: w1481 -> [_ w1519]
                  tunnel: w1479 -> [w1484 w1518]
                  tunnel: w1480 -> [_ w1517]
                  tunnel: w1478 -> [_ w1516]
